vi "RotationRig.vi"() -> ()   [LabVIEW 2010]
panel:
  in  "Yaw Step Size":i32(ring)=2 items=["1.0", "1/16", "1", "1/4", "1/2"]
  in  "Pitch Step Size":i32(ring)=2 items=["1.0", "1/16", "1", "1/4", "1/2"]
  in  "Min/Max Yaw":i32
  in  "Min/Max Pitch":i32
  in  "VISA resource name":refnum<visa-resource-name>="COM1"
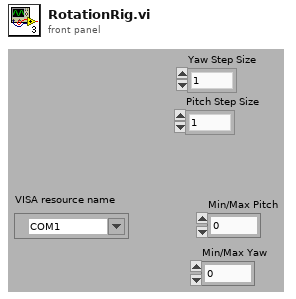
[diagram p1: front panel]
types:
  T1 = enum16{"open", "replace", "create", "open or create", "replace or create", "replace or create with confirmation"}
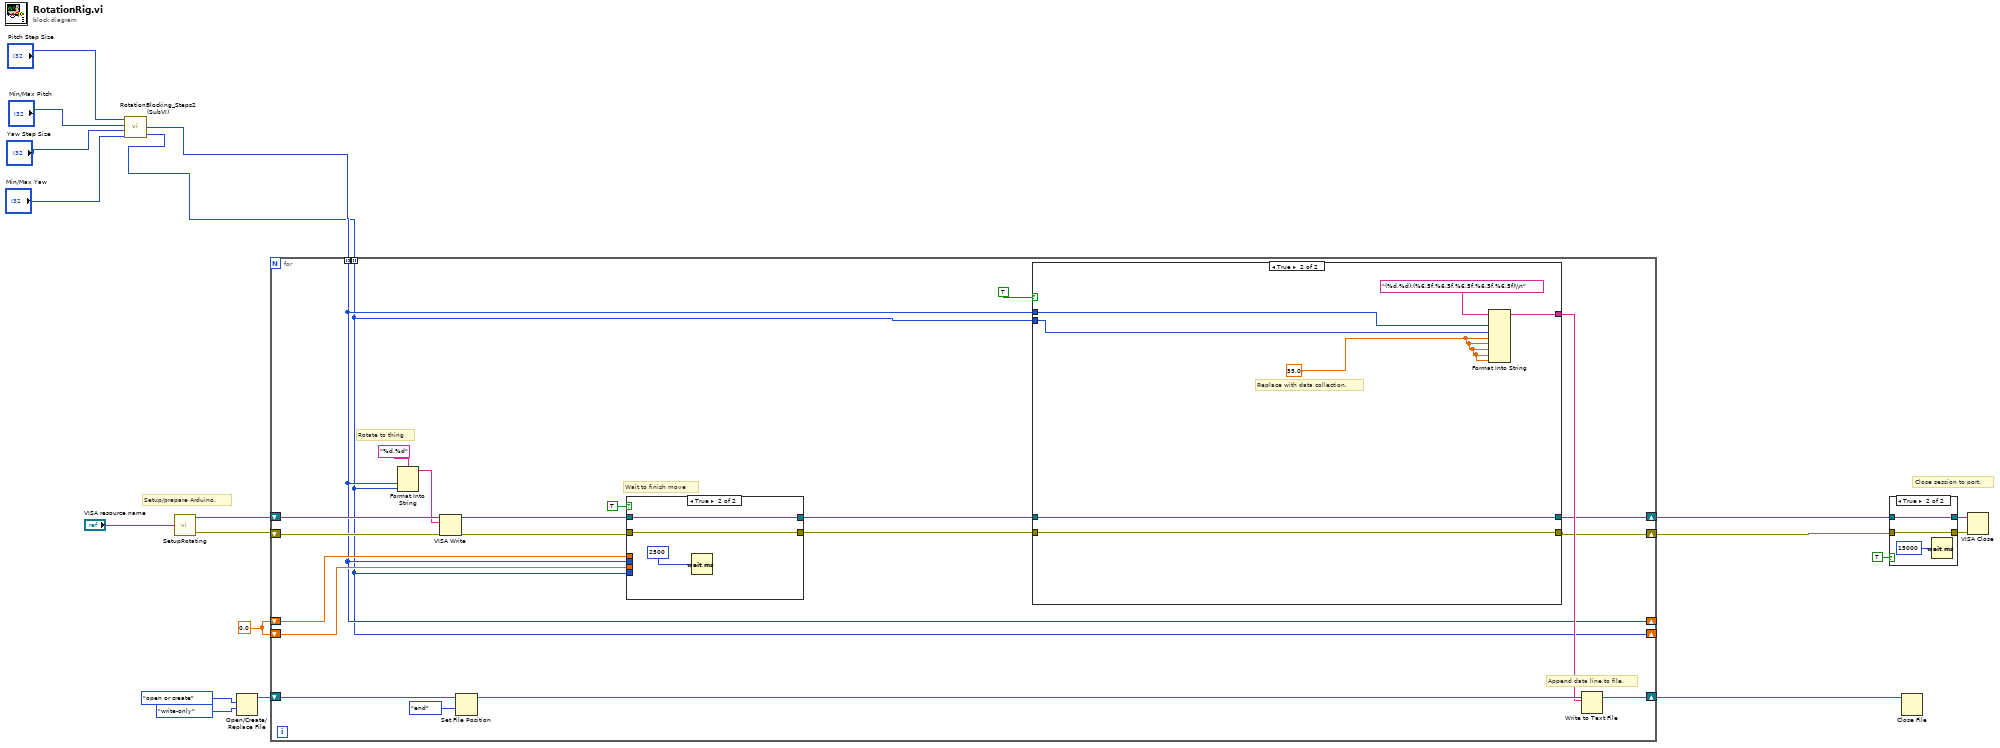
[diagram p0: block diagram]
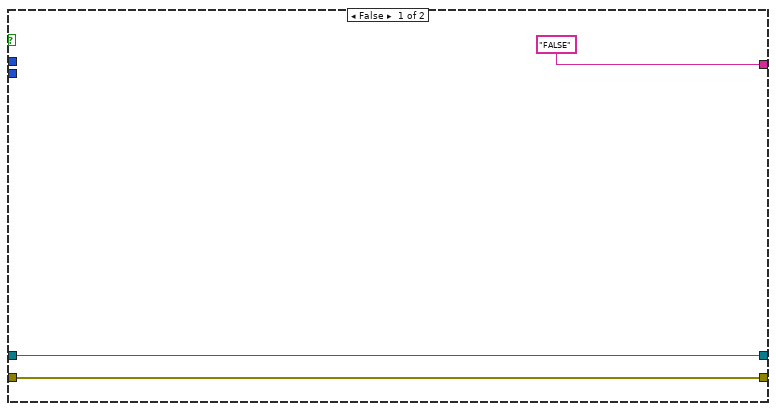
[diagram p2: hidden frame]
diagram:
  w10 = 0.0
  # "Setup/prepare Arduino."
  # "Close session to port."
  n1 = call "RotationBlocking_Steps2 (SubVI).vi"("Min/Max Yaw Steps"="Min/Max Yaw", "Yaw Step Amount"="Yaw Step Size", "Min/Max Pitch Steps"="Min/Max Pitch", "Pitch Step Amount"="Pitch Step Size") -> ("Yaw Array"=w1:i32[], "Pitch Array"=w2:i32[])  [unwired: 1 out]
  n2 = call "SetupRotating.vi"("VISA resource name"="VISA resource name") -> ("error out"=w12:errorcluster, "VISA resource name out"=w13:refnum<visa-resource-name>)
  n3 = Open/Create/Replace File(operation (0:open)=T1."open or create", access (0:read/write)=enum16{"read/write", "read-only", "write-only"}."write-only") -> (refnum out=w15:refnum<file>)  [unwired: 4 in, 2 out]
  n4 = for {
    tunnel: w2 -> [w27] mode=indexing
    tunnel: w1 -> [w26] mode=indexing
    shift-right: [w25] -> w9
    shift-left: w13 -> [w40]
    shift-right: [w23] -> w8
    shift-left: w12 -> [w39]
    shift-right: [w33] -> w7
    shift-left: w15 -> [w36]
    shift-right: [w27] -> _
    shift-left: w10 -> [w32]
    shift-right: [w26] -> _
    shift-left: w10 -> [w31]
    # "Append data line to file."
    # "Wait to finish move"
    # "Rotate to thing"
    n5 = Format Into String(format string="%d,%d" ("string to write 4"), w27, w26) -> (resulting string=w37:string)  [unwired: 2 in, 1 out]
    n6 = VISA Write(VISA resource name=w40, write buffer=w37, error in (no error)=w39) -> (VISA resource name out=w30:refnum<visa-resource-name>, error out=w29:errorcluster)  [unwired: 1 out]
    n7 = Set File Position(refnum=w36, from (0:start)=enum16{"start", "end", "current", ""}."end" ("operation (0:open)")) -> (refnum out=w34:refnum<file>)  [unwired: 2 in, 1 out]
    n8 = case shown="True" TRUE ("write") {
      tunnel: [w52 w55] -> w24
      tunnel: [w51 w54] -> w21
      tunnel: w30 -> [w51 w54]
      tunnel: w29 -> [w52 w55]
      tunnel: w32 -> [_ _]
      tunnel: w31 -> [_ _]
      tunnel: w27 -> [_ _]
      tunnel: w26 -> [_ _]
      frame False {
      }
      frame True {
        n9 = Wait (ms)(milliseconds to wait=2500) -> ()  [unwired: 1 out]
      }
    }
    n10 = case shown="True" TRUE ("write") {
      tunnel: ["FALSE" ("string to write 4") w50] -> w28
      tunnel: w27 -> [_ w48]
      tunnel: w26 -> [_ w47]
      tunnel: [w42 w46] -> w25
      tunnel: w21 -> [w42 w46]
      tunnel: w24 -> [w41 w45]
      tunnel: [w41 w45] -> w23
      frame False {
      }
      frame True {
        w44 = 55.0
        # "Replace with data collection."
        n11 = Format Into String(initial string="(%d,%d);(%6.5f,%6.5f,%6.5f,%6.5f,%6.5f)\\n" ("string to write 4"), w48, w47, w44, w44, w44, w44, w44) -> (resulting string=w50:string)  [unwired: 2 in, 1 out]
      }
    }
    n12 = Write to Text File(file (use dialog)=w34, text=w28) -> (refnum out=w33:refnum<file>)  [unwired: 2 in, 2 out]
  }
  n13 = case shown="True" TRUE ("write") {
    tunnel: [w56 w59] -> w18
    tunnel: [w57 w58] -> w17
    tunnel: w9 -> [w57 w58]
    tunnel: w8 -> [w56 w59]
    frame False {
    }
    frame True {
      n14 = Wait (ms)(milliseconds to wait=u32 15000) -> ()  [unwired: 1 out]
    }
  }
  n15 = Close File(refnum=w7) -> ()  [unwired: 1 in, 2 out]
  n16 = VISA Close(VISA resource name=w17, error in (no error)=w18) -> ()  [unwired: 1 out]
